vi "MISC Get MAC Addresses.vi"(11 "error in (no error)":errorcluster) -> (4 "MAC Addresses":string[](array[string]), 8 "MAC Address Table":string[][](table), 15 "error out":errorcluster)   [LabVIEW 2011]
panel:
  out "ip config Response":string
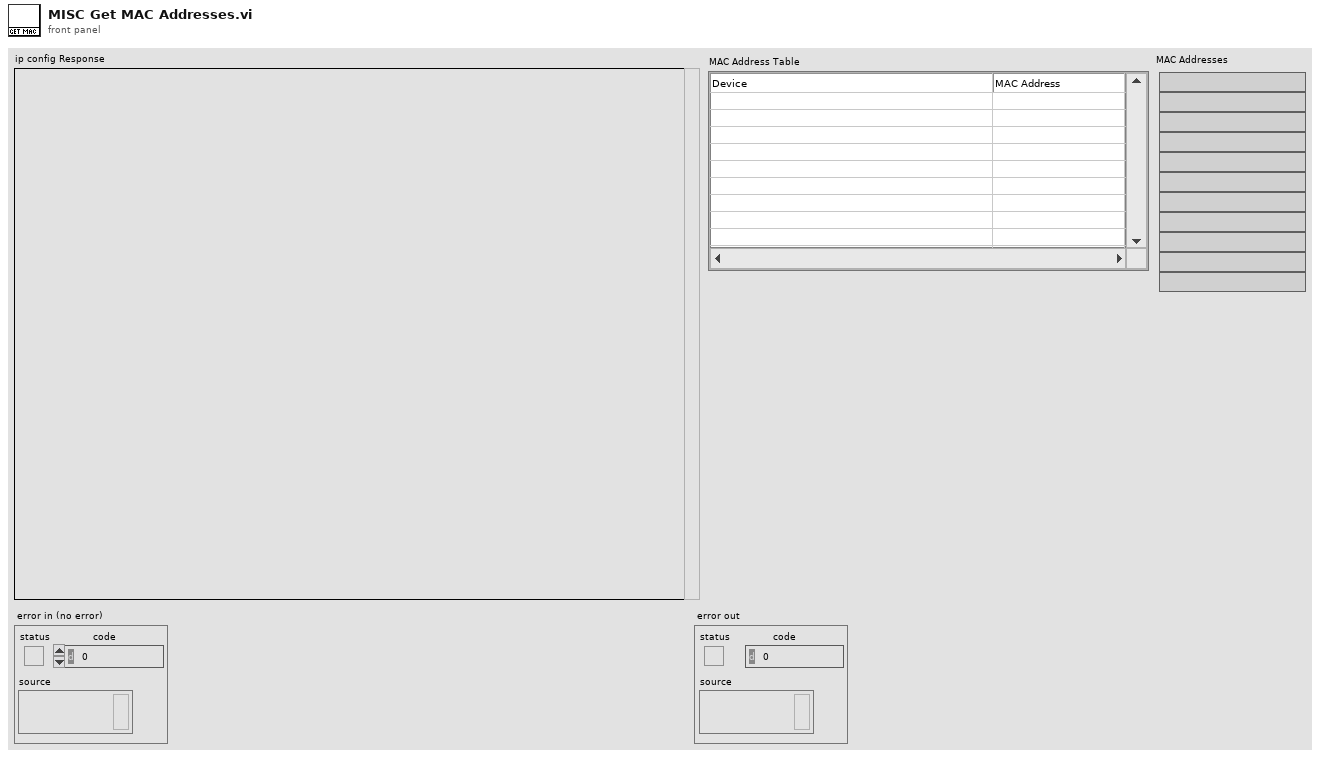
[diagram p1: front panel]
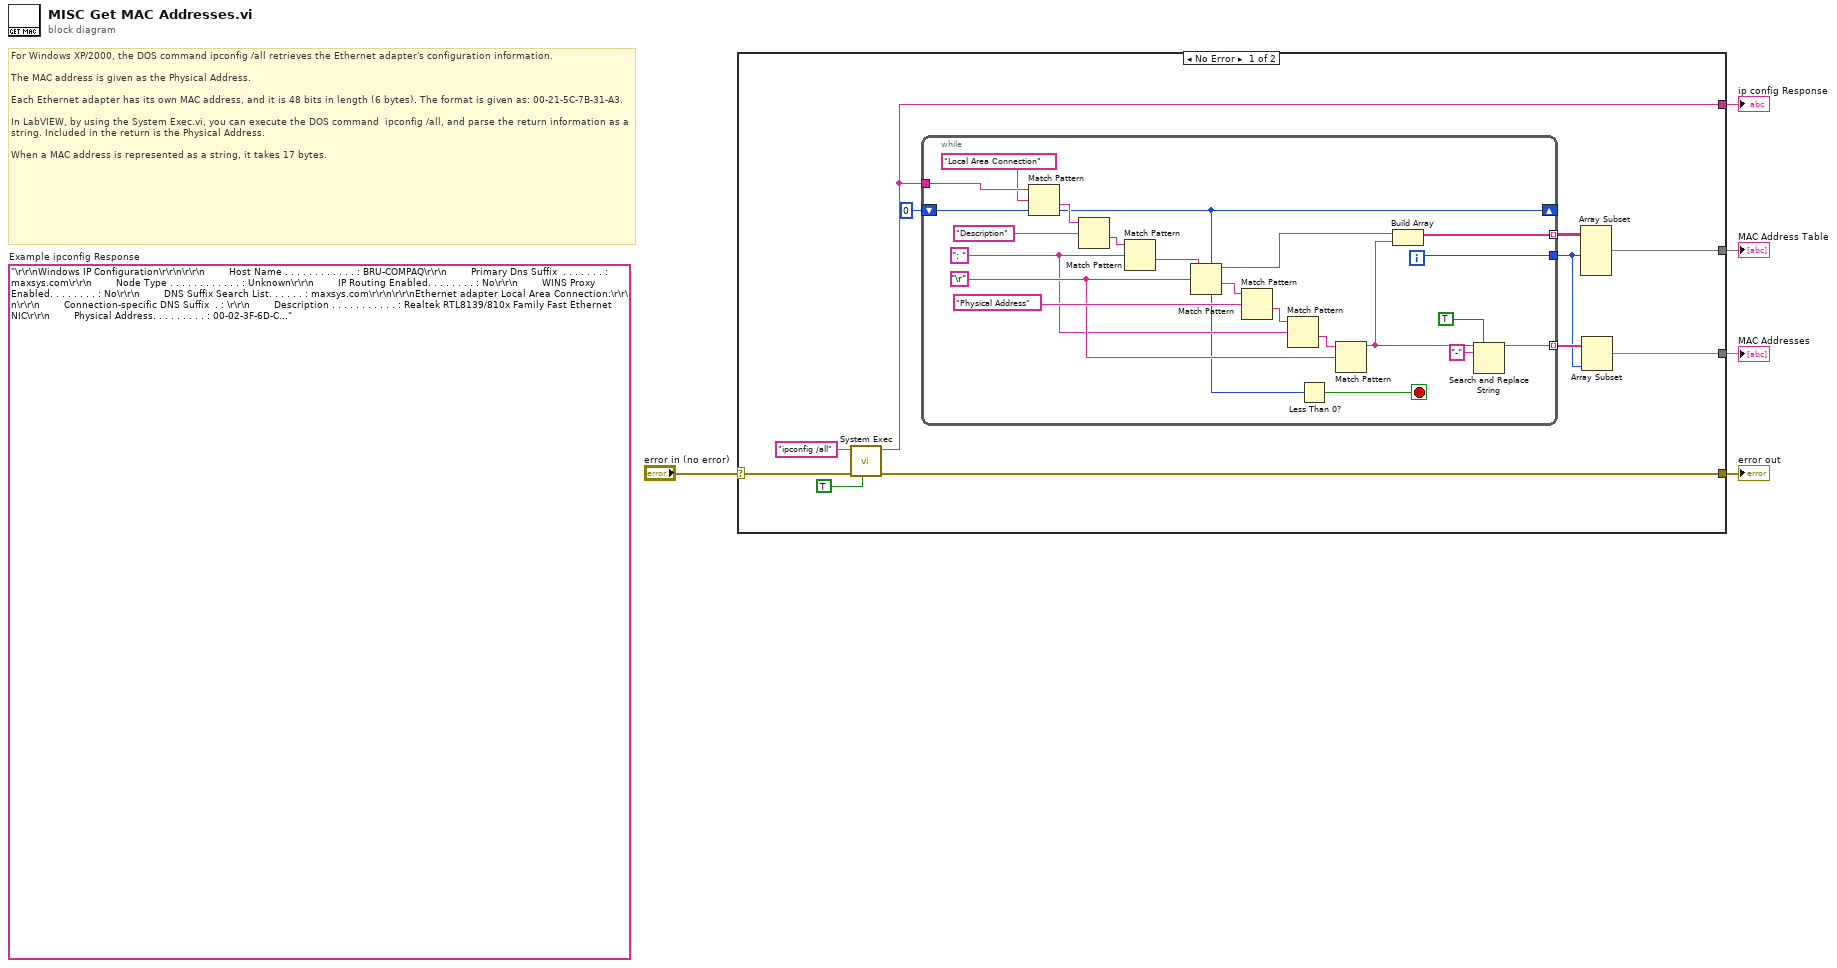
[diagram p0: block diagram]
diagram:
  (unwired) "\r\r\nWindows IP Configuration\r\r\n\r\r\n        Host Name . . . . . . . . . . . . : BRU-COMPAQ\r\r\n        Primary Dns Suffix  . . . . . . . : maxsys.com\r\r\n        Node Type . . . . . . . . . . . . : Unknown\r\r\n        IP Routing Enabled. . . . . . . . : No\r\r\n        WINS Proxy Enabled. . . . . . . . : No\r\r\n        DNS Suffix Search List. . . . . . : maxsys.com\r\r\n\r\r\nEthernet adapter Local Area Connection:\r\r\n\r\r\n        Connection-specific DNS Suffix  . : \r\r\n        Description . . . . . . . . . . . : Realtek RTL8139/810x Family Fast Ethernet NIC\r\r\n        Physical Address. . . . . . . . . : 00-02-3F-6D-C9-AF\r\r\n        Dhcp Enabled. . . . . . . . . . . : No\r\r\n        IP Address. . . . . . . . . . . . : 223.223.223.45\r\r\n        Subnet Mask . . . . . . . . . . . : 255.255.255.0\r\r\n        Default Gateway . . . . . . . . . : 223.223.223.151\r\r\n        DNS Servers . . . . . . . . . . . : 207.182.224.10\r\r\n                                            206.126.128.2\r\r\n\r\r\nEthernet adapter Wireless Network Connection:\r\r\n\r\r\n        Media State . . . . . . . . . . . : Media disconnected\r\r\n        Description . . . . . . . . . . . : Broadcom 802.11b/g WLAN\r\r\n        Physical Address. . . . . . . . . : 00-90-4B-4F-CA-0C\r\r\n\r\r\nEthernet adapter Bluetooth Network Connection:\r\r\n\r\r\n        Media State . . . . . . . . . . . : Media disconnected\r\r\n        Description . . . . . . . . . . . : Bluetooth Device (Personal Area Network)\r\r\n        Physical Address. . . . . . . . . : 00-10-60-D3-5E-E4\r\r\n"  # Example ipconfig Response
  # "For Windows XP/2000, the DOS command ipconfig /all retrieves the Ethernet adapter's configuration information. \n\nThe MAC address is given as the Physical Address. \n\nEach Ethernet adapter has its own MAC address, and it is 48 bits in length (6 bytes). The format is given as: 00-21-5C-7B-31-A3.\n \nIn LabVIEW, by using the System Exec.vi, you can execute the DOS command  ipconfig /all, and parse the return information as a string. Included in the return is the Physical Address. \n\nWhen a MAC address is represented as a string, it takes 17 bytes."
  n1 = case shown="No Error" "error in (no error)" {
    selector: "error in (no error)" -> [w7 _]
    tunnel: [w14 _] -> w5
    tunnel: [w11 _] -> w4
    tunnel: [w6 _] -> w3
    tunnel: [w8 _] -> w2
    frame No Error {
      n2 = call <vilib>:"System Exec.vi"("run minimized? (F)"=TRUE, "error in (no error)"=w7, "command line"="ipconfig /all") -> ("error out"=w8:errorcluster, "standard output"=w14:string)  [unwired: 3 in, 4 out]
      n3 = while {
        tunnel: w14 -> [w38]
        shift-right: [w25] -> _
        shift-left: 0 ("offset past match") -> [w27]
        tunnel: [w22] -> w12 mode=indexing
        tunnel: [w21] -> w9
        tunnel: [w19] -> w10 mode=indexing
        i -> [w21]
        stop <- w24 stop-if-true
        w30 = "\r"
        w26 = ": " ("regular expression")
        n4 = Match Pattern(string=w38, regular expression="Local Area Connection", offset (0)=w27) -> (after substring=w36:string, offset past match=w25:i32)  [unwired: 2 out]
        n5 = Match Pattern(string=w36, regular expression="Description") -> (after substring=w34:string)  [unwired: 4 out]
        n6 = Match Pattern(string=w34, regular expression=w26) -> (after substring=w32:string)  [unwired: 4 out]
        n7 = Match Pattern(string=w32, regular expression=w30) -> (before substring=w23:string, after substring=w31:string)  [unwired: 3 out]
        n8 = Match Pattern(string=w31, regular expression="Physical Address") -> (after substring=w28:string)  [unwired: 4 out]
        n9 = Match Pattern(string=w28, regular expression=w26) -> (after substring=w29:string)  [unwired: 4 out]
        n10 = Less Than 0?(x=w25) -> (x < 0?=w24:bool)
        n11 = Match Pattern(string=w29, regular expression=w30) -> (before substring=w20:string)  [unwired: 4 out]
        n12 = Build Array(w23, w20) -> (w22:string[])
        n13 = Search and Replace String(replace all?=TRUE ("replace all? (F)"), input string=w20, search string="-") -> (result string=w19:string)  [unwired: 1 in, 7 out]
      }
      n14 = Array Subset(array=w12, length (row)=w9) -> (w11:string[][])  [unwired: 3 in]
      n15 = Array Subset(array=w10, length=w9) -> (w6:string[])  [unwired: 1 in]
    }
    frame Error {
    }
  }
  "ip config Response" <- w5
  "MAC Address Table" <- w4
  "MAC Addresses" <- w3
  "error out" <- w2
